vi "binary_cut_out.vi"() -> ()   [LabVIEW 2017]
panel:
  in  "Save":bool
  out "Is OK?":bool
  in  "Stop":bool
  in  "Cut":bool
  out "Waveform Graph 2":waveform(dbl)(graph)
  in  "Length of Cuts in Days":i32=10
  in  "Start of Cut":timestamp=timestamp(3639852000 s since 1904-01-01)
  out "Waveform Graph":waveform(dbl)(graph)
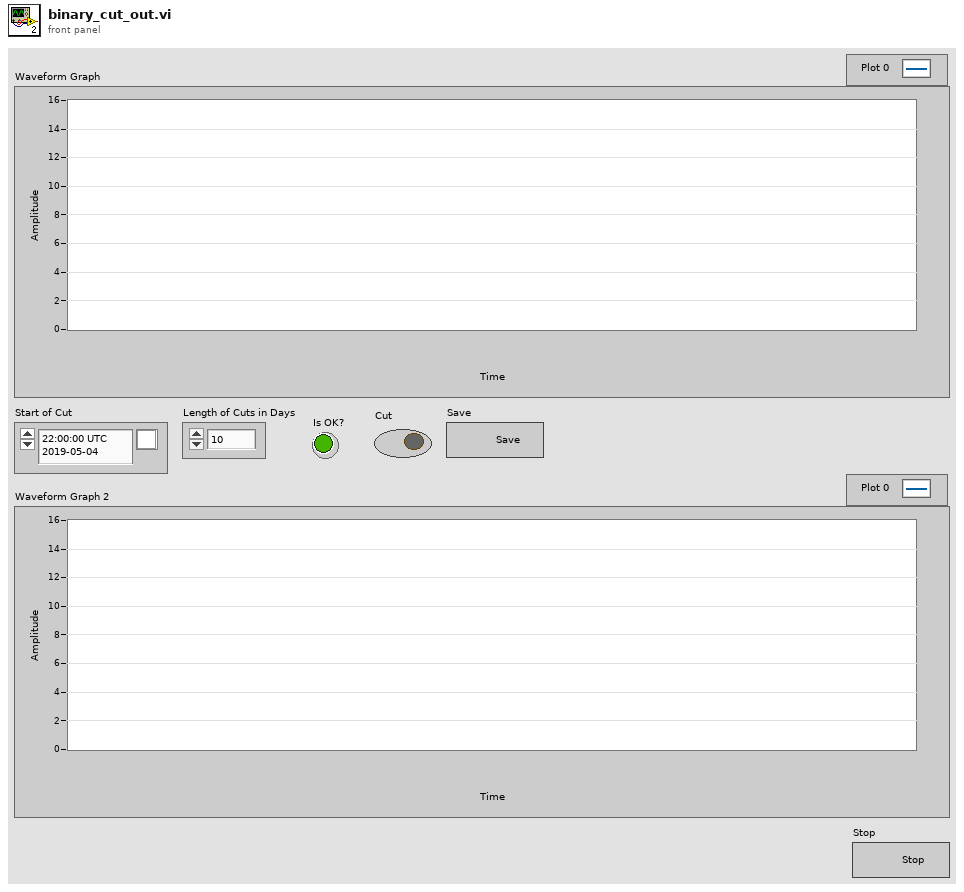
[diagram p1: front panel]
types:
  T1 = typedef "control_all_in_one_package.ctl" = cluster{"memory structure":T2, "actigraph settings":T3, "time informations":T4, "measurement data":T5}
  T2 = typedef "control_memory_structure.ctl" = cluster{"length of metadata [byte]":i32, "length of page [byte]":i32, "length of measurement data on page [byte]":i32, "length of dataset [byte]":i32}
  T3 = typedef "control_measurement_settings.ctl" = cluster{"sampling frequency [Hz]":dbl, "measurement interval [± g]":i32, "high precision?":bool, "number of pages":i32, "rate code":i32, "range code":i32, "id":i32}
  T4 = typedef "control_time_informations.ctl" = cluster{"starting time":timestamp, "ending time":timestamp, "dt[s]":dbl, "sampling rate [Hz]":dbl, "length":dbl}
  T5 = typedef "control_measurement_data.ctl" = cluster{"number of samples per axis":i32, "timestamp array":dbl[], "offset array":dbl[], "x, y, z axis data":waveform(dbl)[], "normalised magnitude of acceleartion vectors":waveform(dbl), "calibration coefficients":T6, "statistics":T7, "battery voltage":waveform(dbl), "magnitude of acceleartion vectors":waveform(dbl)}
  T6 = typedef "control_calibration_coefficients.ctl" = cluster{"Sx":dbl, "Ox":dbl, "Sy":dbl, "Oy":dbl, "Sz":dbl, "Oz":dbl}
  T7 = typedef "control_statistics.ctl" = cluster{"mean of x axis acceleration":dbl, "standard devation of x axis acceleration":dbl, "mean of y axis acceleration":dbl, "standard devation of y axis acceleration":dbl, "mean of z axis acceleration":dbl, "standard devation of z axis acceleration":dbl, "mean of normalised magnitude of acceleration":dbl, "standard devation of normalised magnitude of acceleration":dbl}
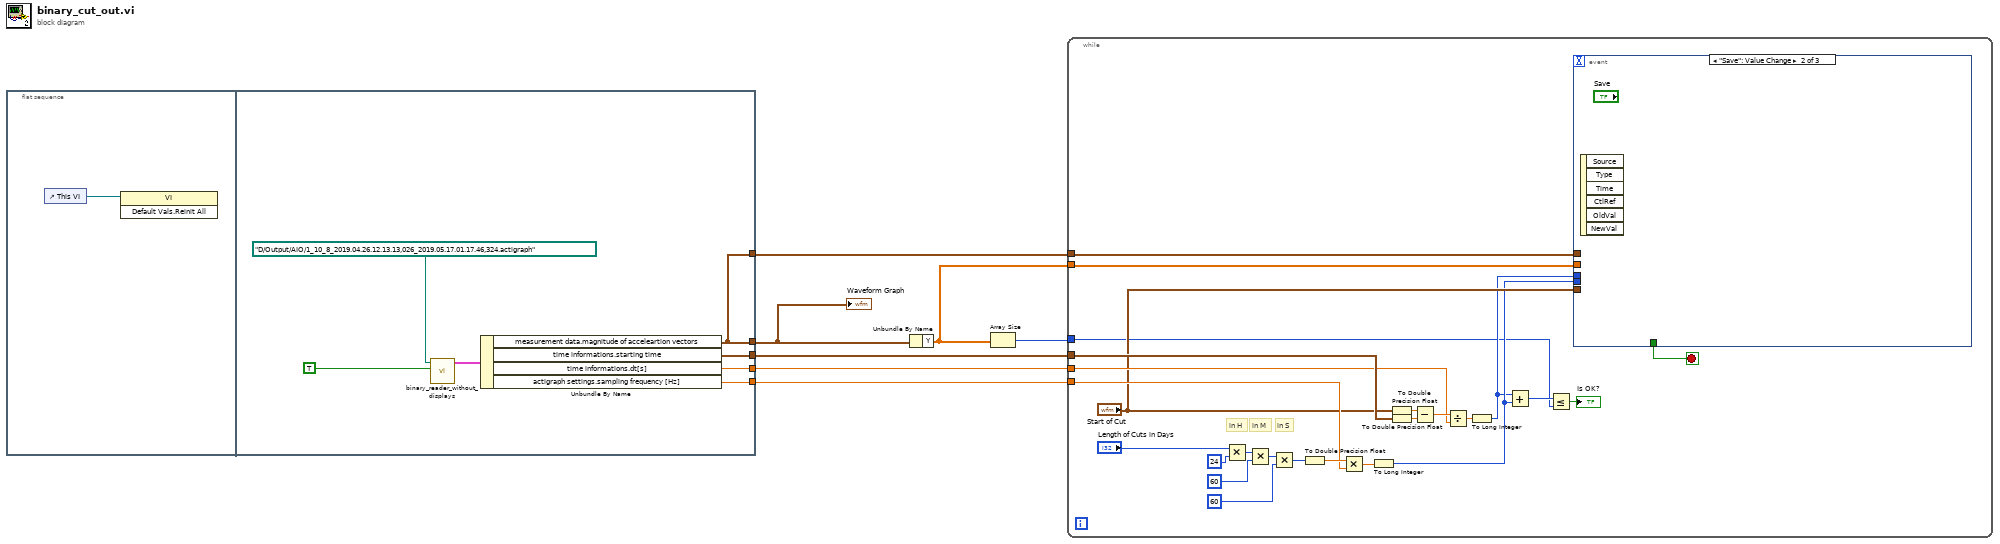
[diagram p0: block diagram]
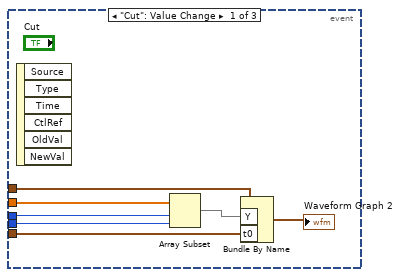
[diagram p2: hidden frame]
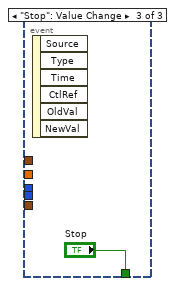
[diagram p3: hidden frame]
diagram:
  n1 = flat-sequence {
    tunnel: [w12] -> w7
    tunnel: [w11] -> w6
    tunnel: [w10] -> w5
    tunnel: [w9] -> w4
    tunnel: [w9] -> w2
    frame #0 {
      n2 = control-ref of="This VI"() -> (w8:refnum<vi>)
      n3 = invoke class="VI" method="Default Vals.Reinit All"(reference=w8) -> ()  [unwired: 2 in, 3 out]
    }
    frame #1 {
      n4 = call "binary_reader_without_displays.vi"("are calibration coefficients\n available in the binary file?"=TRUE ("are calibration coefficients\n available in the binary file?"), "path to binary file"=path "D:/Output/AIO/1_10_8_2019.04.26.12.13.13,026_2019.05.17.01.17.46,324.actigraph") -> ("all in one package"=w13:T1)  [unwired: 7 in, 1 out]
      n5 = Unbundle By Name(w13) -> ("measurement data.magnitude of acceleartion vectors"=w9:waveform(dbl), "time informations.starting time"=w12:timestamp, "time informations.dt[s]"=w11:dbl, "actigraph settings.sampling frequency [Hz]"=w10:dbl)
    }
  }
  n6 = Unbundle By Name(w4) -> ("Y"=w1:dbl[])
  n7 = Array Size(array=w1) -> (size(s)=w3:i32)
  n8 = while {
    tunnel: w7 -> [w39]
    tunnel: w6 -> [w36]
    tunnel: w5 -> [w26]
    tunnel: w3 -> [w19]
    tunnel: w2 -> [w18]
    tunnel: w1 -> [w17]
    stop <- w16 stop-if-true
    # "in S"
    # "in M"
    # "in H"
    n9 = Multiply(x="Length of Cuts in Days", y=24) -> (x*y=w32:i32)
    n10 = Multiply(x=w32, y=60) -> (x*y=w30:i32)
    n11 = Multiply(x=w30, y=60) -> (x*y=w28:i32)
    n12 = To Double Precision Float(number=w28) -> (double precision float=w27:dbl)
    n13 = Multiply(x=w27, y=w26) -> (x*y=w25:dbl)
    n14 = To Long Integer(number=w25) -> (32bit integer=w22:i32)
    n15 = To Double Precision Float(number="Start of Cut") -> (double precision float=w40:dbl)
    n16 = To Double Precision Float(number=w39) -> (double precision float=w38:dbl)
    n17 = Subtract(x=w40, y=w38) -> (x-y=w37:dbl)
    n18 = Divide(x=w37, y=w36) -> (x/y=w35:dbl)
    n19 = To Long Integer(number=w35) -> (32bit integer=w21:i32)
    n20 = Add(x=w21, y=w22) -> (x+y=w20:i32)
    n21 = Less Or Equal?(x=w20, y=w19) -> (x <= y?=→"Is OK?":bool)
    n22 = event shown="[1] \"Save\": Value Change" {
      selector: _ -> [_ _ _]
      dyn-events: _ -> [_ _ _]
      timeout: _ -> [_ _ _]
      tunnel: w18 -> [w45 _ _]
      tunnel: "Start of Cut" -> [w44 _ _]
      tunnel: w17 -> [w43 _ _]
      tunnel: w21 -> [w42 _ _]
      tunnel: w22 -> [w41 _ _]
      tunnel: [_ _ "Stop"] -> w16
      event "Cut": Value Change {
        n23 = event-data() -> ()  [unwired: 1 in, 6 out]
        n24 = Array Subset(array=w43, index=w42, length=w41) -> (w46:dbl[])
        n25 = Bundle By Name(cluster=w45, "Y"=w46, "t0"=w44) -> (→"Waveform Graph 2":waveform(dbl))
      }
      event "Save": Value Change {
        n26 = event-data() -> ()  [unwired: 1 in, 6 out]
      }
      event "Stop": Value Change {
        n27 = event-data() -> ()  [unwired: 1 in, 6 out]
      }
    }
  }
  "Waveform Graph" <- w4
